vi "checkTemperatureSettled.vi"(8 "error in (no error)":errorcluster, 11 "Model in":refnum<class "Model.lvclass">) -> (0 "error out":errorcluster, 2 "tempSettledIsTrue":bool, 3 "Model out":refnum<class "Model.lvclass">)   [LabVIEW 2013, in "Model.lvclass"]
uses:
  Model.lvclass
  Model.lvclass/Model.ctl
  UserEvents/UserEvents.lvclass/UserEvents.ctl
  ApplicationElements/TestMonitor/TestMonitor.lvclass/TestMonitor.ctl
  ApplicationElements/TestMonitor/TestMonitor.lvclass
  UserEvents/UserEvents.lvclass
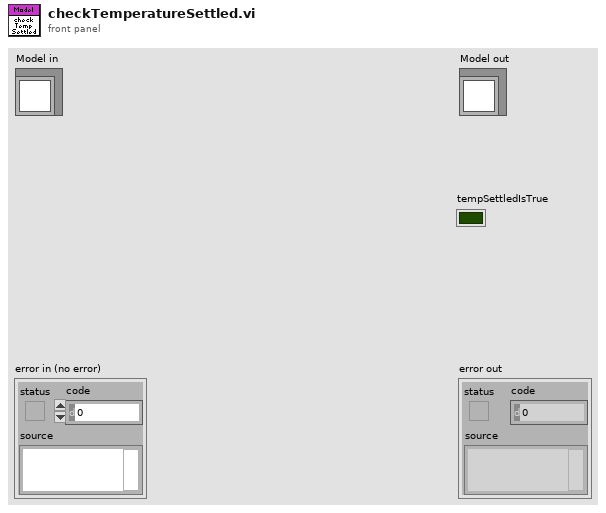
[diagram p1: front panel]
types:
  T1 = typedef "AITDTTypedefs.lvlib/PubDataEvents.ctl" = cluster{"State":refnum<user-event>, "ErrorCode":refnum<user-event>, "OutputData":refnum<user-event>, "InputData":refnum<user-event>, "TestStatus":refnum<user-event>, "LogPath":refnum<user-event>, "TemperatureSetpointRequest":refnum<user-event>, "TemperatureSettling":refnum<user-event>, "WaitTimeStatus":refnum<user-event>}
  T2 = typedef "AITDTTypedefs.lvlib/TemperatureSettling.ctl" = cluster{"Temperature Measured":dbl[unit], "TemperatureSettledIsTrue":bool, "Required":cluster{"Sample Size Rqd":u16, "StDev":dbl[unit]}, "Measured":cluster{"StDev Msd":dbl[unit], "Sample Size Msd":u16}}
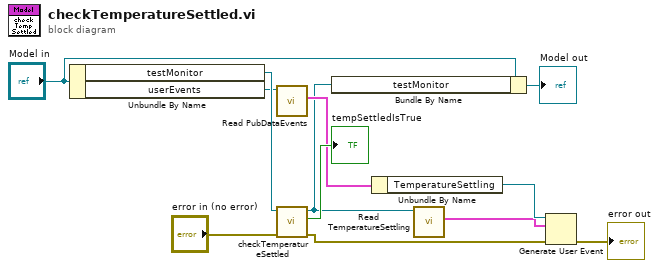
[diagram p0: block diagram]
diagram:
  n1 = Unbundle By Name("Model in") -> ("testMonitor"=w12:refnum<class "TestMonitor.lvclass">, "userEvents"=w7:refnum<class "UserEvents.lvclass">)
  n2 = call "Read PubDataEvents.vi"("UserEvents in"=w7) -> ("PubDataEvents"=w6:T1)  [unwired: 9 in, 1 out]
  n3 = call "checkTemperatureSettled.vi"("error in (no error)"="error in (no error)", "TestMonitor in"=w12) -> ("error out"=w2:errorcluster, "temperatureSettledIsTrue"=→"tempSettledIsTrue":bool, "TestMonitor out"=w3:refnum<class "TestMonitor.lvclass">)  [unwired: 7 in]
  n4 = Bundle By Name(cluster="Model in", "testMonitor"=w3) -> (→"Model out":refnum<class "Model.lvclass">)
  n5 = Unbundle By Name(w6) -> ("TemperatureSettling"=w5:refnum<user-event>)
  n6 = call "Read TemperatureSettling.vi"("TestMonitor in"=w3) -> ("TemperatureSettling"=w4:T2)  [unwired: 9 in, 1 out]
  n7 = Generate User Event(user event=w5, event data cluster=w4, error in=w2) -> (error out=→"error out":errorcluster)  [unwired: 1 in, 1 out]
